vi "Convert Data Type code to string - Single Input.vi"(8 "Error In":errorcluster, 11 "Type code":i32) -> (0 "Error Out":errorcluster, 2 "Type string":string)   [LabVIEW 2014]
doc: "<B>Copyright</B>: (c) MHWirth 2015.\n\nThis VI converts the array of data types (string) to array of data type codes (int32). \n\n<B>Defined Type Code</B>:\nUnknown/Undefined type returns -1. \nCode 1. Boolean\nCode 2 to 5. Int8/16/32/64\nCode 6 to 9. UInt8/16/32/64\nCode 10. Double\nCode 11. Single-precision\nCode 12. String\nCode 13 to 24. 1D array of xxx\nCode 25 to 36. 2D array of xxx"
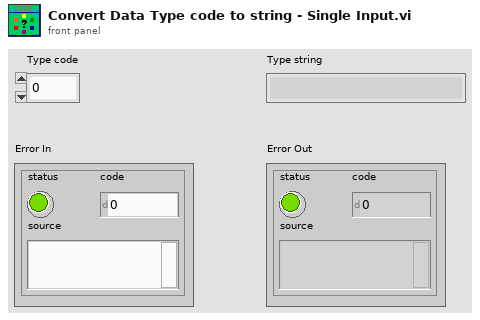
[diagram p1: front panel]
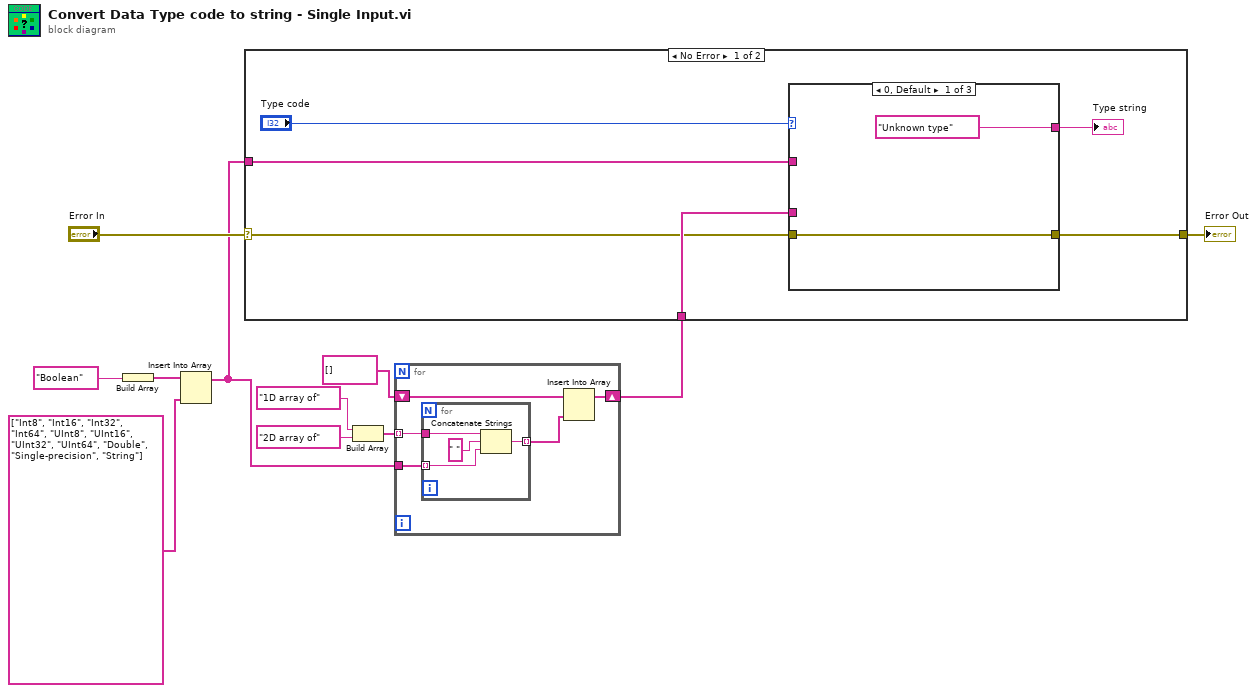
[diagram p0: block diagram]
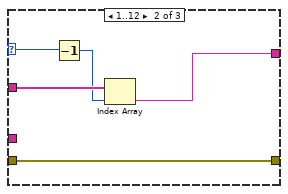
[diagram p2: hidden frame]
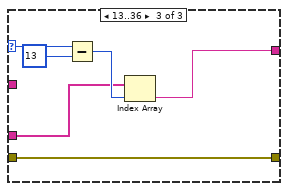
[diagram p3: hidden frame]
diagram:
  n1 = Build Array("Boolean") -> (w5:string[])
  n2 = Insert Into Array(array=w5, new element=string[] ["Int8", "Int16", "Int32", "Int64", "UInt8", "UInt16", "UInt32", "UInt64", "Double", "Single-precision", "String"]) -> (w3:string[])  [unwired: 1 in]
  n3 = Build Array("1D array of", "2D array of") -> (w7:string[])
  n4 = for {
    tunnel: w7 -> [w16] mode=indexing
    shift-right: [w13] -> w1
    shift-left: string[] [] -> [w15]
    tunnel: w3 -> [w12]
    n5 = for {
      tunnel: w16 -> [w20]
      tunnel: w12 -> [w18] mode=indexing
      tunnel: [w17] -> w14 mode=indexing
      n6 = Concatenate Strings(w20, " ", w18) -> (w17:string)
    }
    n7 = Insert Into Array(array=w15, new element=w14) -> (w13:string[])  [unwired: 1 in]
  }
  n8 = case shown="No Error" "Error In" {
    selector: "Error In" -> [w21 w40]
    tunnel: [w22 w40] -> w10
    tunnel: w3 -> [w24 _]
    tunnel: w1 -> [w23 _]
    frame No Error {
      n9 = case shown="0, Default" "Type code" {
        selector: "Type code" -> [_ w33 w38]
        tunnel: ["Unknown type" w30 w39] -> w25
        tunnel: w24 -> [_ w32 _]
        tunnel: w23 -> [_ _ w34]
        tunnel: [w27 w29 w35] -> w22
        tunnel: w21 -> [w27 w29 w35]
        frame 0, Default {
        }
        frame 1..12 {
          n10 = Decrement(x=w33) -> (x-1=w31:i32)
          n11 = Index Array(array=w32, index=w31) -> (element=w30:string)
        }
        frame 13..36 {
          n12 = Subtract(x=w38, y=13) -> (x-y=w36:i32)
          n13 = Index Array(array=w34, index=w36) -> (element=w39:string)
        }
      }
      "Type string" <- w25
    }
    frame Error {
    }
  }
  "Error Out" <- w10
